vi "mxwScript_API_XMLWireToNodeByIndex.vi"(8 "error in (no error)":errorcluster, 10 "terminalIndex":u32, 11 "nodeLabel":string) -> (0 "error out":errorcluster, 3 "encoded connector name":string)   [LabVIEW 2020]
doc: "Create encoded control name for connecting to a terminal on a generic node instead of to a control terminal. Terminal is specified by index.\n\nThis encoding works for both connected to and connected from terminals."
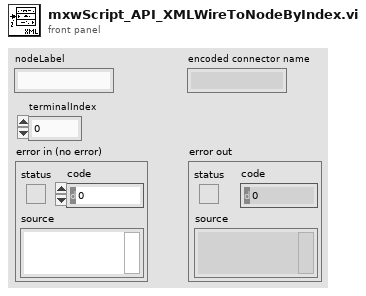
[diagram p1: front panel]
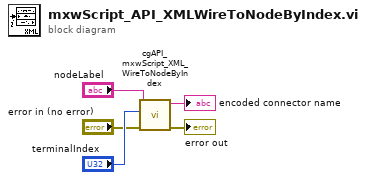
[diagram p0: block diagram]
diagram:
  n1 = call "cgAPI_mxwScript_XML_WireToNodeByIndex.vi"("error in (no error)"="error in (no error)", "terminalIndex"="terminalIndex", "nodeLabel"="nodeLabel") -> ("error out"=→"error out":errorcluster, "encoded connector name"=→"encoded connector name":string)  [unwired: 7 out]
